vi "RTDRead.vi"(6 "Numeric 15":dbl, 8 "Numeric 14":dbl, 9 "Numeric 13":dbl, 10 "Numeric 12":dbl, 11 "Array in":dbl[](array[numeric])) -> (3 "Array out":dbl[](array[numeric]))   [LabVIEW 2017]
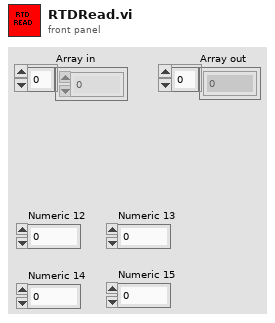
[diagram p1: front panel]
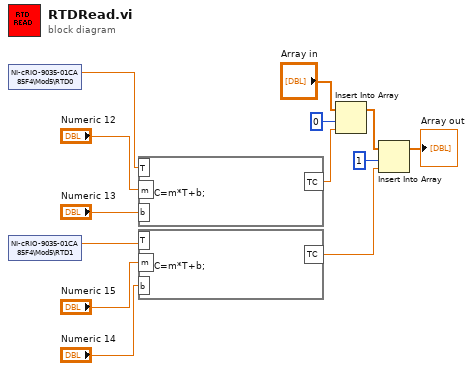
[diagram p0: block diagram]
diagram:
  n1 = shared-variable "NI-cRIO-9035-01CA85F4\\Mod5\\RTD0"() -> (w8:dbl)  [unwired: 1 in, 1 out]
  n2 = shared-variable "NI-cRIO-9035-01CA85F4\\Mod5\\RTD1"() -> (w1:dbl)  [unwired: 1 in, 1 out]
  n3 = formula code="TC=m*T+b;"("T"=w8, "m"="Numeric 12", "b"="Numeric 13") -> ("TC"=w7:dbl)
  n4 = formula code="TC=m*T+b;"("T"=w1, "m"="Numeric 15", "b"="Numeric 14") -> ("TC"=w2:dbl)
  n5 = Insert Into Array(array="Array in", index=0, new element=w7) -> (w11:dbl[])
  n6 = Insert Into Array(array=w11, index=1, new element=w2) -> (→"Array out":dbl[])
